vi "CRC5 EPC.vi"(8 "error in (no error)":errorcluster, 11 "data":u8[](array[numeric])) -> (0 "error out":errorcluster, 3 "crc":u8[](array[numeric]))   [LabVIEW 2023]
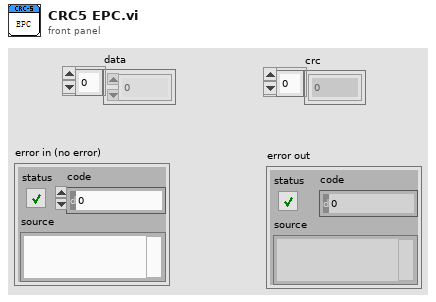
[diagram p1: front panel]
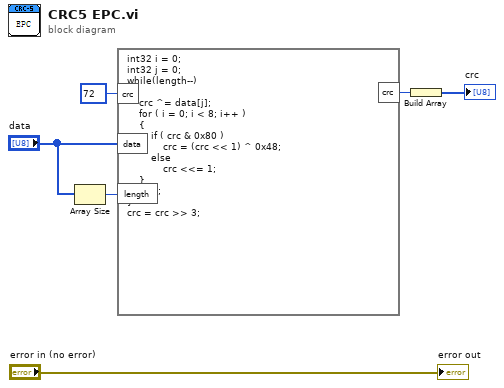
[diagram p0: block diagram]
diagram:
  n1 = Array Size(array="data") -> (size(s)=w6:i32)
  n2 = formula code="int32 i = 0;\nint32 j = 0;\nwhile(length--)\n{\n    crc ^= data[j]; \n    for ( i = 0; i < 8; i++ )\n    {\n        if ( crc & 0x80 )\n            crc = (crc << 1) ^ 0x48;\n        else\n            crc <<= 1;\n    }\n    j++;\n}\ncrc = crc >> 3;"("data"="data", "length"=w6, "crc"=u8 72) -> ("crc"=w4:u8)
  n3 = Build Array(w4) -> (→"crc":u8[])
  "error out" <- "error in (no error)"
